vi "CANOpen_Initialize VS BiDirectional Data Refs.vi"(7 "Name":string, 8 "error in (no error)":errorcluster, 10 "Hardware Output Refs":T1[](array[typedef]) format="%.0x", 11 "Device Ref":T1 format="%.0x") -> (0 "error out":errorcluster, 2 "Data References":T2 {"Hardware Output"."Channel Pairs"."Chan Refs" format="%.0x"}, 3 "Device Ref out":T1=18446744073709551615 format="%.0x")   [LabVIEW 2021, in "CANOpen Addon Engine.lvlib"]
uses:
  CANOpen Addon Engine.lvlib
  CANOpen_VS Bidirectional Data Refs.ctl
  <vilib>/NI VeriStand/Custom Device API/Data Reference.ctl
  <vilib>/NI VeriStand/Custom Device API/Custom Device Item Ref.ctl
  <vilib>/NI VeriStand/Custom Device API/Data Access Type.ctl
  <vilib>/NI VeriStand/Custom Device API/Custom Device API.lvlib
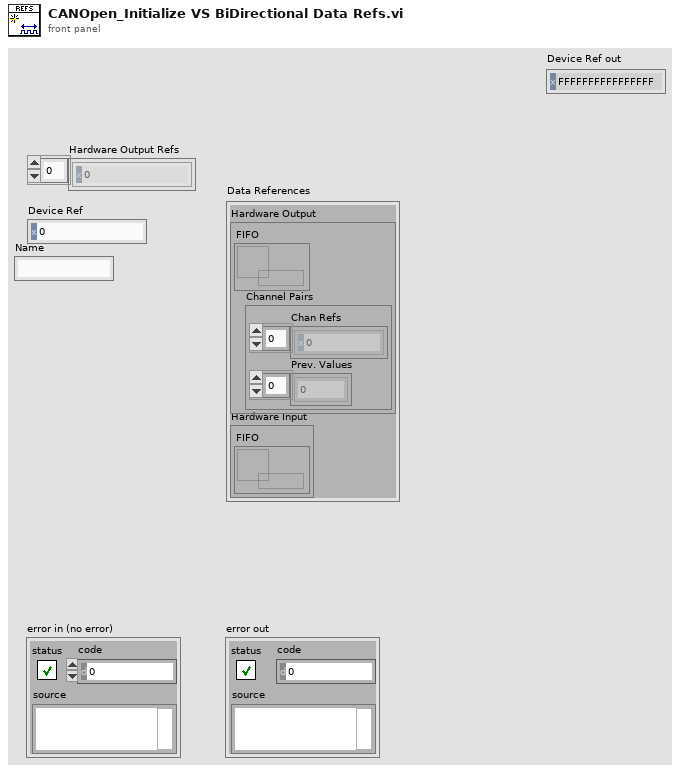
[diagram p1: front panel]
types:
  T1 = typedef "Custom Device API.lvlib/Custom Device Item Ref.ctl" = u64
  T2 = typedef "CANOpen Addon Engine.lvlib/CANOpen_VS Bidirectional Data Refs.ctl" = cluster{"Hardware Output":cluster{"FIFO":refnum<k33>, "Channel Pairs":cluster{"Chan Refs":T3[], "Prev. Values":dbl[]}}, "Hardware Input":cluster{"FIFO":refnum<k33>}}
  T3 = typedef "Custom Device API.lvlib/Data Reference.ctl" = i32
  T4 = cluster{"read mode":enum16{"polling", "blocking"}, "write mode":enum16{"polling", "blocking"}}
  T5 = typedef "Custom Device API.lvlib/Data Access Type.ctl" = enum16{"Read", "Write"}
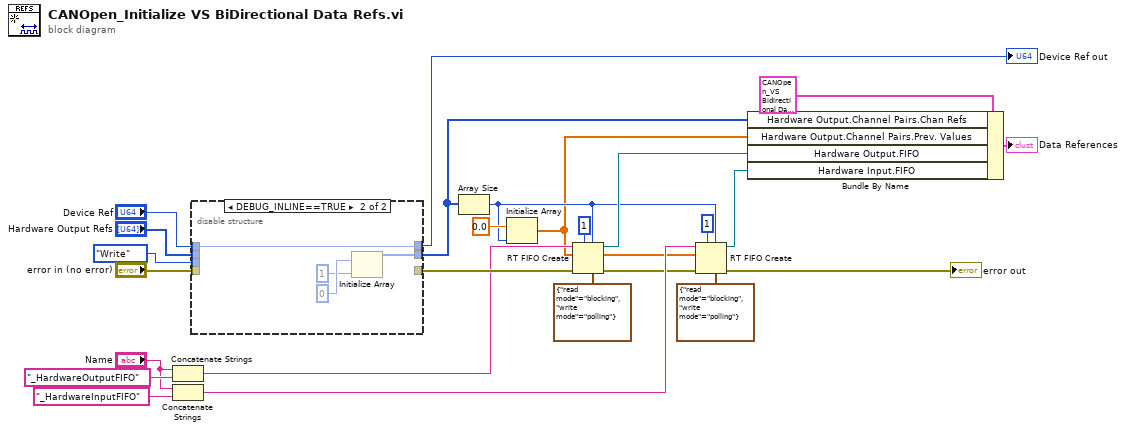
[diagram p0: block diagram]
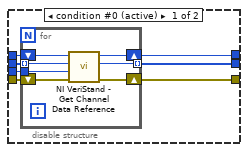
[diagram p2: hidden frame]
diagram:
  n1 = Concatenate Strings("Name", "_HardwareOutputFIFO" ("string")) -> (w7:string)
  n2 = Concatenate Strings("Name", "_HardwareInputFIFO" ("string")) -> (w6:string)
  n3 = disable-structure shown="DEBUG_INLINE==TRUE" {
    disable-tunnel: [w32 w41] -> w23
    disable-tunnel: [w31 _] -> w16
    disable-tunnel: Data_Access_Type."Write" ("Access") -> [w30 _]
    disable-tunnel: "Hardware Output Refs" -> [w29 _]
    disable-tunnel: "Device Ref" -> [w28 w43]
    disable-tunnel: "error in (no error)" -> [w27 _]
    disable-tunnel: [w26 w43] -> w3
    frame condition #0 (active) {
      n4 = for {
        tunnel: w29 -> [w35] mode=indexing
        tunnel: w30 -> [w34]
        shift-right: [w37] -> w31
        shift-left: w27 -> [w38]
        shift-right: [w39] -> w26
        shift-left: w28 -> [w36]
        tunnel: [w33] -> w32 mode=indexing
        n5 = call <vilib>:"NI VeriStand - Get Channel Data Reference.vi"("error in (no error)"=w38, "Access"=w34, "Channel Ref in"=w35, "Device Ref in"=w36) -> ("error out"=w37:errorcluster, "Channel Data Reference"=w33:T3, "Device Ref out"=w39:T1)  [unwired: 5 in]
      }
    }
    frame condition #1 {
      n6 = Initialize Array(T3 0 ("Channel Data Reference"), 1 ("dimension size")) -> (w41:T3[])
    }
  }
  "Device Ref out" <- w3
  n7 = Array Size(array=w23) -> (size(s)=w4:i32)
  n8 = Initialize Array(0.0 ("element"), w4) -> (w2:dbl[])
  n9 = RT FIFO Create(0:w7, 1:w2, 3:w16, 4:u32 1 ("size (10)"), 6:w4, 7:T4 {"read mode"=enum."blocking", "write mode"=enum."polling"} ("r/w modes (polling,polling)")) -> (8:w22:refnum<k33>, 11:w1:errorcluster)  [unwired: 2 in, 1 out]
  n10 = RT FIFO Create(0:w6, 1:w2, 3:w1, 4:u32 1 ("size (10)"), 6:w4, 7:T4 {"read mode"=enum."blocking", "write mode"=enum."polling"} ("r/w modes (polling,polling)")) -> (8:w24:refnum<k33>, 11:→"error out":errorcluster)  [unwired: 2 in, 1 out]
  n11 = Bundle By Name(cluster=T2 {"Hardware Output"={"FIFO"=refnum, "Channel Pairs"={"Chan Refs"=[], "Prev. Values"=[]}}, "Hardware Input"={"FIFO"=refnum}} ("Data References"), "Hardware Output.Channel Pairs.Chan Refs"=w23, "Hardware Output.Channel Pairs.Prev. Values"=w2, "Hardware Output.FIFO"=w22, "Hardware Input.FIFO"=w24) -> (→"Data References":T2)
